vi "Default Instrument Setup.vi"(8 "error in (no error)":errorcluster, 11 "VISA resource name":refnum<visa-resource-name>) -> (0 "error out":errorcluster, 3 "VISA resource name out":refnum<visa-resource-name>)   [LabVIEW 2018, in "Lake Shore 372.lvlib"]
doc: "Sends a default command string to the instrument whenever a new VISA session is opened, or the instrument is reset. This VI is intended to be used as a subVI for the LSCI 370 Initialize and LSCI 370 Reset VI's. Altering this VI could cause these two VI's to operate incorrectly."
uses:
  Lake Shore 372.lvlib
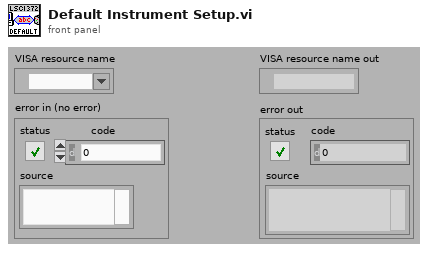
[diagram p1: front panel]
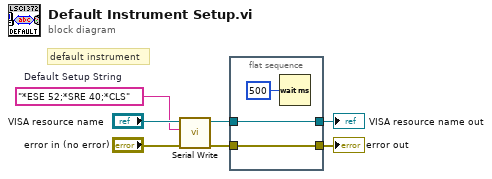
[diagram p0: block diagram]
diagram:
  w3 = "*ESE 52;*SRE 40;*CLS"  # Default Setup String
  # "default instrument"
  n1 = call "Serial Write.vi"("error in (no error)"="error in (no error)", "Write Buffer (\"\")"=w3, "VISA resource name"="VISA resource name") -> ("error out"=w6:errorcluster, "VISA resource name out"=w5:refnum<visa-resource-name>)  [unwired: 6 in, 1 out]
  n2 = flat-sequence {
    tunnel: w6 -> [w10]
    tunnel: [w10] -> w1
    tunnel: w5 -> [w9]
    tunnel: [w9] -> w4
    frame #0 {
      n3 = Wait (ms)(milliseconds to wait=u32 500) -> ()  [unwired: 1 out]
    }
  }
  "VISA resource name out" <- w4
  "error out" <- w1
